vi "Identify.vi"(3 "error in":errorcluster, 5 "VISA arduino in":refnum<visa-resource-name>) -> (0 "error out":errorcluster, 1 "identification":string, 2 "VISA arduino out":refnum<visa-resource-name>)   [LabVIEW 2021]
uses:
  Delay_Global.vi
  <vilib>/Utility/error.llb/Error Cluster From Error Code.vi
  <vilib>/ErrorRing/Error Ring.xnode
panel:
  out "delay":u32
  # "Private"
  # "Public"
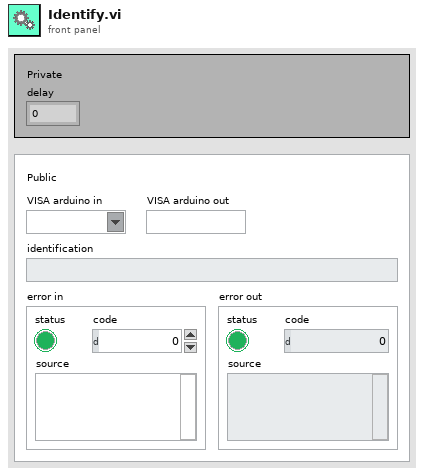
[diagram p1: front panel]
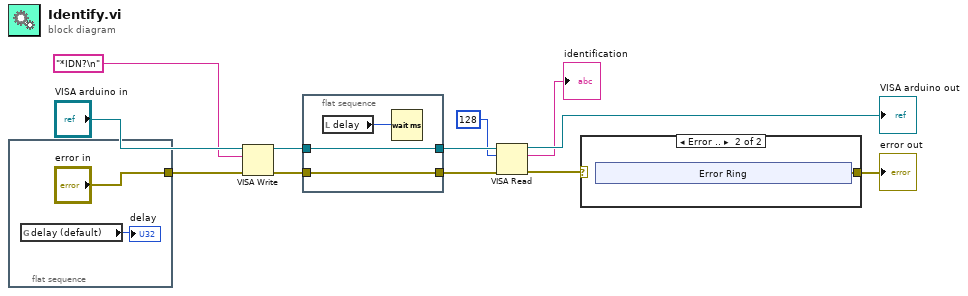
[diagram p0: block diagram]
diagram:
  n1 = flat-sequence {
    tunnel: ["error in"] -> w8
    frame #0 {
      n2 = global read "Delay_Global.vi" "delay (default)"() -> (→"delay":u32)
    }
  }
  n3 = VISA Write(VISA resource name="VISA arduino in", write buffer="*IDN?\n", error in (no error)=w8) -> (VISA resource name out=w12:refnum<visa-resource-name>, error out=w11:errorcluster)  [unwired: 1 out]
  n4 = flat-sequence {
    tunnel: [w17] -> w5
    tunnel: w12 -> [w17]
    tunnel: [w16] -> w6
    tunnel: w11 -> [w16]
    frame #0 {
      n5 = local read "delay"() -> (w15:u32)
      n6 = Wait (ms)(milliseconds to wait=w15) -> ()  [unwired: 1 out]
    }
  }
  n7 = VISA Read(VISA resource name=w5, byte count=u32 128, error in (no error)=w6) -> (VISA resource name out=→"VISA arduino out":refnum<visa-resource-name>, read buffer=→"identification":string, error out=w3:errorcluster)  [unwired: 1 out]
  n8 = case shown="Error .." w3 {
    selector: w3 -> [w18 _]
    tunnel: [w18 w19] -> w10
    frame No Error {
    }
    frame Error {
      n9 = xnode "Error Ring"() -> ("error out"=w19:errorcluster)
    }
  }
  "error out" <- w10
